vi "NaN_extracter.vi"(11 "Array 1":dbl[](array[numeric])) -> (3 "Array 2":dbl[](array[numeric]))   [LabVIEW 2014]
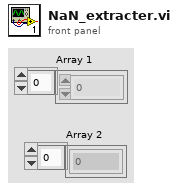
[diagram p1: front panel]
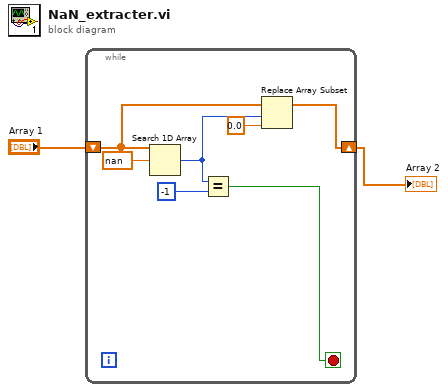
[diagram p0: block diagram]
diagram:
  n1 = while {
    shift-right: [w3] -> w1
    shift-left: "Array 1" -> [w6]
    stop <- w7 stop-if-true
    n2 = Search 1D Array(1D array=w6, element=nan) -> (index of element=w5:i32)  [unwired: 1 in]
    n3 = Equal?(x=w5, y=-1) -> (x = y?=w7:bool)
    n4 = Replace Array Subset(array=w6, new element=0.0 ("new element/subarray"), index=w5) -> (w3:dbl[])
  }
  "Array 2" <- w1
